vi "RepeatedLines.vi"() -> ()   [LabVIEW 2016]
uses:
  <vilib>/Utility/file.llb/Read Delimited Spreadsheet (DBL).vi
panel:
  in  "Line Widths [mm]":dbl[](array[numeric]) format="%#_13g"
  in  "Line Separations [mm]":dbl[][](array[numeric]) format="%#_13g"
  in  "First Line Width [mm]":dbl
  in  "N Lines [mm]":i32
  in  "Stereo Angle":dbl format="%#_13g"
  out "Stave Angle":dbl format="%#_13g"
  in  "Line Separation [mm]":dbl[](array[numeric]) format="%#_13g"
  in  "Line Width [mm]":dbl format="%#_13g"
  in  "ShiftToGlue [mm]":dbl[](array[numeric])
  in  "Nth Module":dbl
  in  "Axis Speeds":T1={"X [mm/s]"=25.0, "Y [mm/s]"=25.0, "Z [mm/s]"=25.0}
  out "Virtual Stave Map":path
  in  "Calibration Directory":path
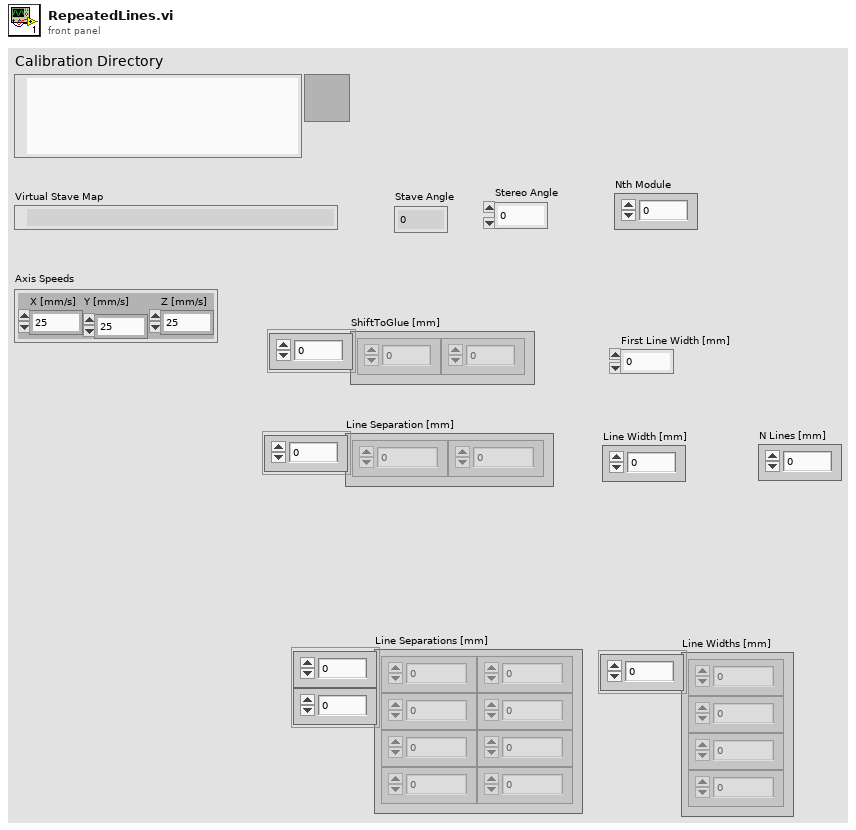
[diagram p1: front panel]
types:
  T1 = cluster{"X [mm/s]":dbl, "Y [mm/s]":dbl, "Z [mm/s]":dbl}
  T2 = cluster{"Final X":dbl, "Final Y":dbl, "Final Z":dbl}
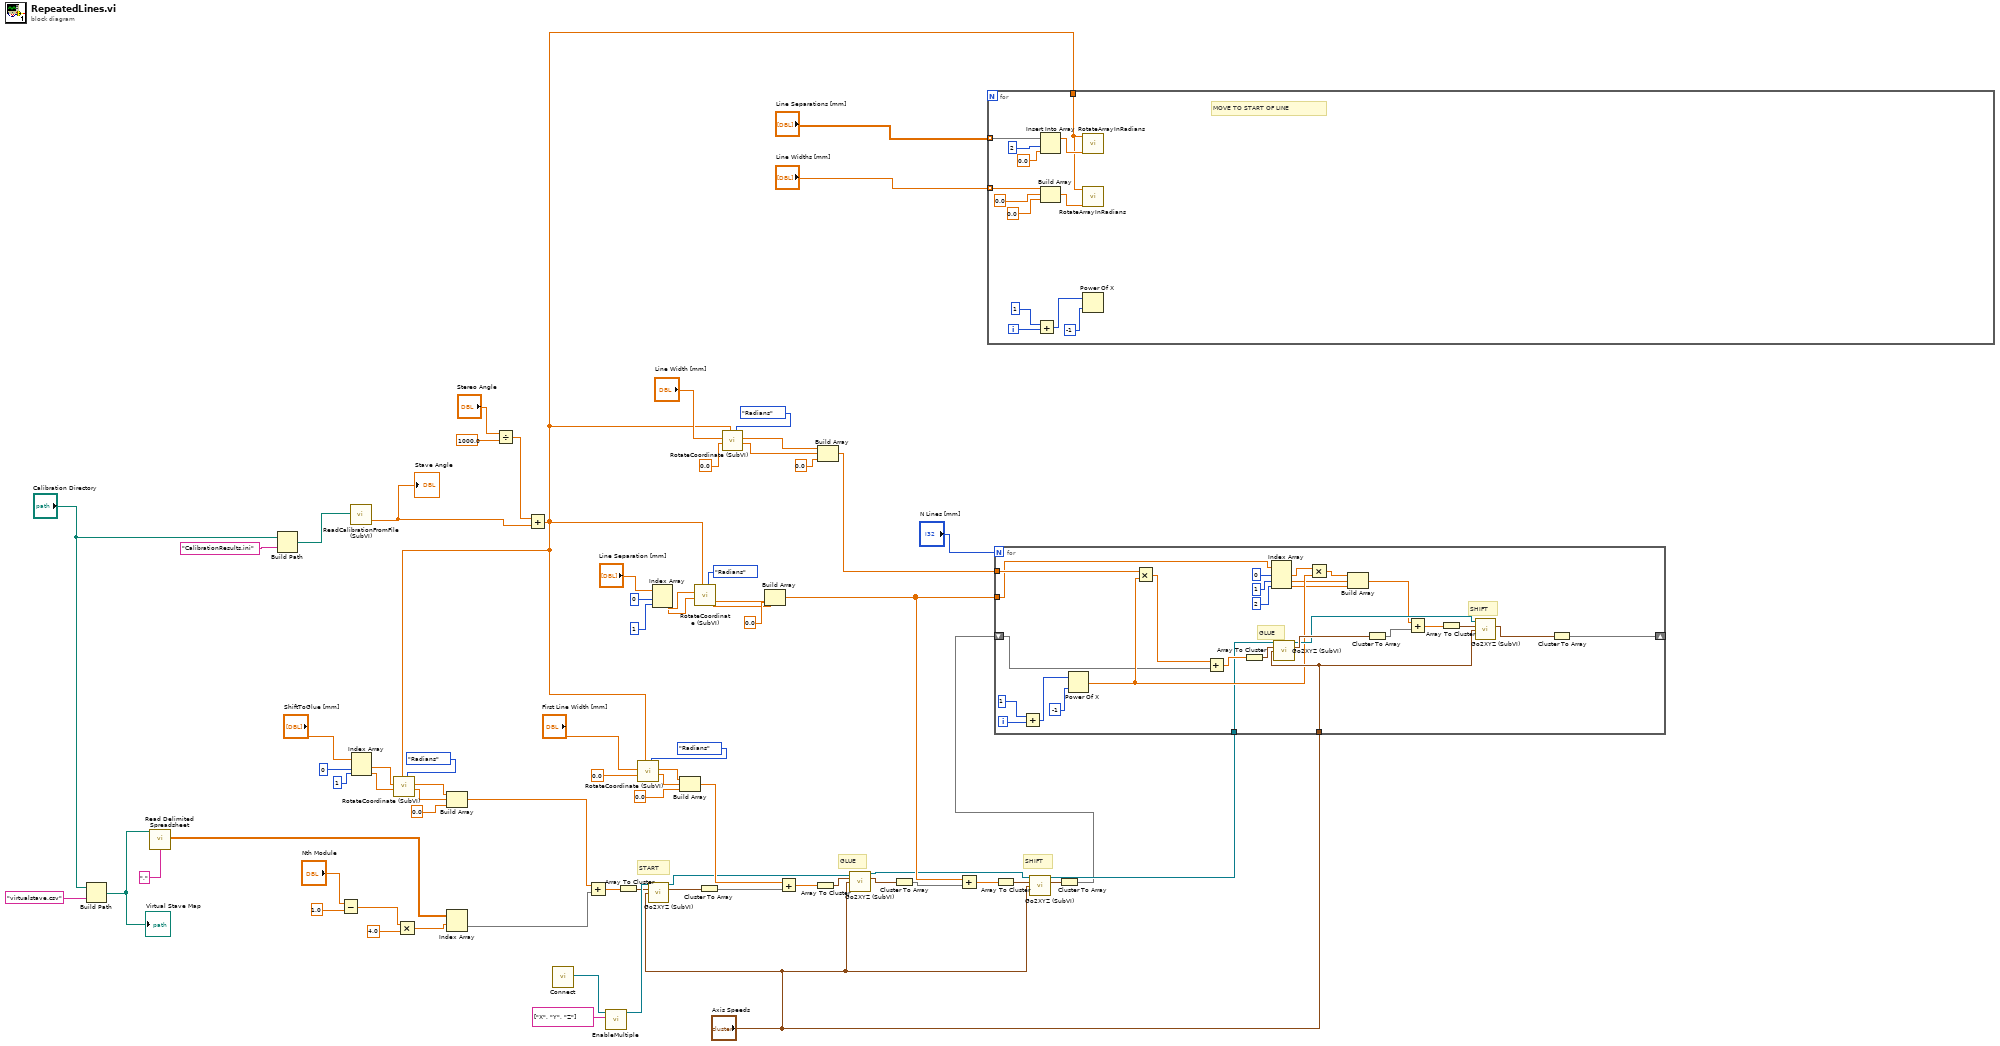
[diagram p0: block diagram]
diagram:
  # "START"
  # "SHIFT"
  # "GLUE"
  n1 = Build Path(base path="Calibration Directory", name or relative path="virtualstave.csv") -> (appended path=w73:path)
  "Virtual Stave Map" <- w73
  n2 = call-poly <vilib>:"Read Delimited Spreadsheet.vi"("file path (dialog if empty)"=w73, "delimiter (\\t)"="," ("delimiter (\\t)")) -> ("all rows"=w66:dbl[][])  [unwired: 8 in, 5 out]
  n3 = Build Path(base path="Calibration Directory", name or relative path="CalibrationResults.ini") -> (appended path=w63:path)
  n4 = Subtract(x="Nth Module", y=1.0) -> (x-y=w69:dbl)
  n5 = call "ReadCalibrationFromFile (SubVI).vi"("Calibration file path"=w63) -> ("Angle"=w60:dbl)  [unwired: 12 in, 6 out]
  "Stave Angle" <- w60
  n6 = Index Array(array="ShiftToGlue [mm]", index #1=0 ("index"), index #2=1 ("index")) -> (element #1=w42:dbl, element #2=w43:dbl)
  n7 = Multiply(x=w69, y=4.0) -> (x*y=w71:dbl)
  n8 = Index Array(array=w66, index (row)=w71) -> (element=w47:dbl[])  [unwired: 1 in]
  n9 = Divide(x="Stereo Angle", y=1000.0) -> (x/y=w57:dbl)
  n10 = Add(x=w57, y=w60) -> (x+y=w1:dbl)
  n11 = call "RotateCoordinate (SubVI).vi"("Units"=enum16{"mrad", "Radians", "Degrees"}."Radians", "Angle"=w1, "y"=w43, "x"=w42) -> ("y'"=w39:dbl, "x'"=w38:dbl)  [unwired: 5 in, 1 out]
  n12 = Build Array(w38, w39, 0.0 ("element")) -> (w40:dbl[])
  n13 = call <vilib>:"Connect.vi"() -> ("controller"=w65:refnum<k24>)  [unwired: 10 in, 1 out]
  n14 = Add(x=w40, y=w47) -> (x+y=w34:dbl[])
  n15 = call "EnableMultiple.vi"("axis names"=string[] ["X", "Y", "Z"] ("Axes Names"), "controller in"=w65) -> ("controller out"=w36:refnum<k24>)  [unwired: 8 in, 1 out]
  n16 = Array To Cluster(array=w34) -> (cluster=w35:cluster{"[0]":dbl, "[1]":dbl, "[2]":dbl})
  n17 = call "RotateCoordinate (SubVI).vi"("Units"=enum16{"mrad", "Radians", "Degrees"}."Radians", "Angle"=w1, "y"=0.0, "x"="First Line Width [mm]") -> ("y'"=w27:dbl, "x'"=w28:dbl)  [unwired: 5 in, 1 out]
  n18 = call "Go2XYZ (SubVI).vi"(".NET Refnum in"=w36, "Go to Coordinates"=w35, "Axis Speeds"="Axis Speeds") -> (".NET Refnum out"=w23:refnum<k24>, "Final Position"=w32:T2)  [unwired: 8 in, 3 out]
  n19 = Index Array(array="Line Separation [mm]", index #1=0 ("index"), index #2=1 ("index")) -> (element #1=w17:dbl, element #2=w16:dbl)
  n20 = Build Array(w28, w27, 0.0 ("element")) -> (w25:dbl[])
  n21 = call "RotateCoordinate (SubVI).vi"("Units"=enum16{"mrad", "Radians", "Degrees"}."Radians", "Angle"=w1, "y"=w16, "x"=w17) -> ("y'"=w49:dbl, "x'"=w48:dbl)  [unwired: 5 in, 1 out]
  n22 = Cluster To Array(cluster=w32) -> (array=w24:dbl[])
  n23 = call "RotateCoordinate (SubVI).vi"("Units"=enum16{"mrad", "Radians", "Degrees"}."Radians", "Angle"=w1, "y"=0.0 ("element"), "x"="Line Width [mm]") -> ("y'"=w51:dbl, "x'"=w52:dbl)  [unwired: 5 in, 1 out]
  n24 = Build Array(w48, w49, 0.0 ("element")) -> (w11:dbl[])
  n25 = Add(x=w25, y=w24) -> (x+y=w22:dbl[])
  n26 = Array To Cluster(array=w22) -> (cluster=w21:cluster{"[0]":dbl, "[1]":dbl, "[2]":dbl})
  n27 = Build Array(w52, w51, 0.0 ("element")) -> (w33:dbl[])
  n28 = call "Go2XYZ (SubVI).vi"(".NET Refnum in"=w23, "Go to Coordinates"=w21, "Axis Speeds"="Axis Speeds") -> (".NET Refnum out"=w7:refnum<k24>, "Final Position"=w13:T2)  [unwired: 8 in, 3 out]
  n29 = Cluster To Array(cluster=w13) -> (array=w12:dbl[])
  n30 = Add(x=w11, y=w12) -> (x+y=w10:dbl[])
  n31 = for {
    tunnel: "Line Separations [mm]" -> [w80] mode=indexing
    tunnel: "Line Widths [mm]" -> [w81] mode=indexing
    tunnel: w1 -> [w75]
    i -> [w85]
    # "MOVE TO START OF LINE"
    n32 = Add(x=1, y=w85) -> (x+y=w84:i32)
    n33 = Insert Into Array(array=w80, index=2, new element=0.0 ("new element/subarray")) -> (w77:dbl[])
    n34 = Build Array(w81, 0.0 ("element"), 0.0 ("element")) -> (w76:dbl[])
    n35 = call "RotateArrayInRadians.vi"("X,Y,Z Input"=w77, "Angle"=w75) -> ()  [unwired: 9 in, 1 out]
    n36 = call "RotateArrayInRadians.vi"("X,Y,Z Input"=w76, "Angle"=w75) -> ()  [unwired: 9 in, 1 out]
    n37 = Power Of X(1:-1 ("x"), 2:w84) -> ()  [unwired: 1 out]
  }
  n38 = Array To Cluster(array=w10) -> (cluster=w9:cluster{"[0]":dbl, "[1]":dbl, "[2]":dbl})
  n39 = call "Go2XYZ (SubVI).vi"(".NET Refnum in"=w7, "Go to Coordinates"=w9, "Axis Speeds"="Axis Speeds") -> (".NET Refnum out"=w6:refnum<k24>, "Final Position"=w5:T2)  [unwired: 8 in, 3 out]
  n40 = Cluster To Array(cluster=w5) -> (array=w4:dbl[])
  n41 = for {
    N: "N Lines [mm]" -> [_]
    tunnel: "Axis Speeds" -> [w106]
    tunnel: w33 -> [w104]
    tunnel: w11 -> [w103]
    shift-right: [w90] -> _
    shift-left: w4 -> [w89]
    tunnel: w6 -> [w88]
    i -> [w92]
    # "SHIFT"
    # "GLUE"
    n42 = Add(x=1, y=w92) -> (x+y=w93:i32)
    n43 = Power Of X(1:-1 ("x"), 2:w93) -> (0:w101:dbl)
    n44 = Multiply(x=w104, y=w101) -> (x*y=w114:dbl[])
    n45 = Add(x=w114, y=w89) -> (x+y=w113:dbl[])
    n46 = Array To Cluster(array=w113) -> (cluster=w112:cluster{"[0]":dbl, "[1]":dbl, "[2]":dbl})
    n47 = Index Array(array=w103, index #1=0 ("index"), index #2=1 ("index"), index #3=2 ("index")) -> (element #1=w100:dbl, element #2=w97:dbl, element #3=w96:dbl)
    n48 = call "Go2XYZ (SubVI).vi"(".NET Refnum in"=w88, "Go to Coordinates"=w112, "Axis Speeds"=w106) -> (".NET Refnum out"=w107:refnum<k24>, "Final Position"=w111:T2)  [unwired: 8 in, 3 out]
    n49 = Multiply(x=w100, y=w101) -> (x*y=w95:dbl)
    n50 = Build Array(w95, w97, w96) -> (w94:dbl[])
    n51 = Cluster To Array(cluster=w111) -> (array=w110:dbl[])
    n52 = Add(x=w94, y=w110) -> (x+y=w109:dbl[])
    n53 = Array To Cluster(array=w109) -> (cluster=w108:cluster{"[0]":dbl, "[1]":dbl, "[2]":dbl})
    n54 = call "Go2XYZ (SubVI).vi"(".NET Refnum in"=w107, "Go to Coordinates"=w108, "Axis Speeds"=w106) -> ("Final Position"=w105:T2)  [unwired: 8 in, 4 out]
    n55 = Cluster To Array(cluster=w105) -> (array=w90:dbl[])
  }
